vi "Tag to Block.vi"(10 "Block Tag":string) -> (2 "Block":string)   [LabVIEW 2022 SP3, in "FlexBlocks Support.lvlib"]
uses:
  FlexBlocks Support.lvlib
  <vilib>/regexp/Match Regular Expression.xnode
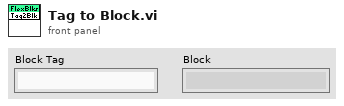
[diagram p1: front panel]
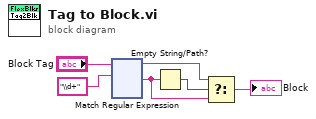
[diagram p0: block diagram]
diagram:
  n1 = xnode "Match Regular Expression"("input string"="Block Tag", "regular expression"="\\d+") -> ("before match"=w3:string, "after match"=w5:string)  [unwired: 4 in, 3 out]
  n2 = Empty String/Path?(string/path=w5) -> (empty?=w4:bool)
  n3 = Select(t=w3, s=w4, f=w5) -> (s? t:f=→"Block":string)
